vi "Get Console Reply(class).vi"(8 "error in (no error)":errorcluster, 11 "EditPanel API in":refnum<class "EditPanel API.lvclass">) -> (0 "error out":errorcluster, 2 "EditPanel API.lvlib:Console Reply.lvclass":refnum<class "Console Reply.lvclass">, 3 "EditPanel API out":refnum<class "EditPanel API.lvclass">)   [LabVIEW 2015, in "EditPanel API.lvlib" / "EditPanel API.lvclass"]
uses:
  EditPanel API.lvclass
  Console Reply/Console Reply/Console Reply.lvclass
  EditPanel API.lvclass/EditPanel API.ctl
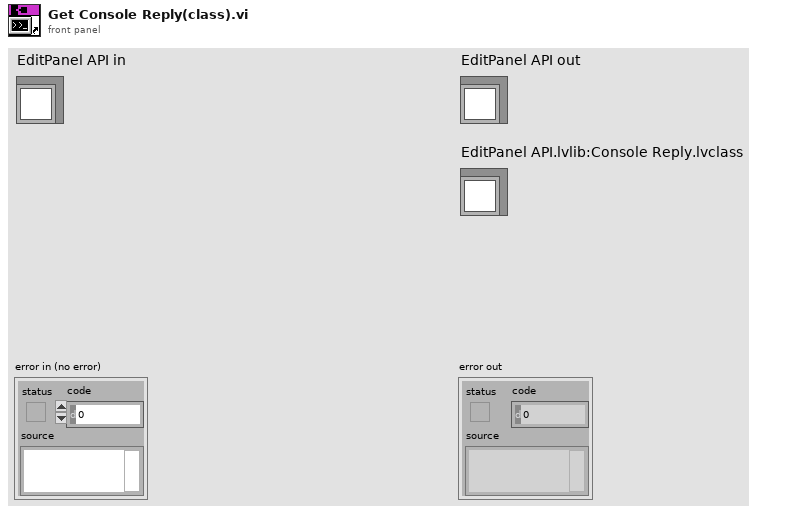
[diagram p1: front panel]
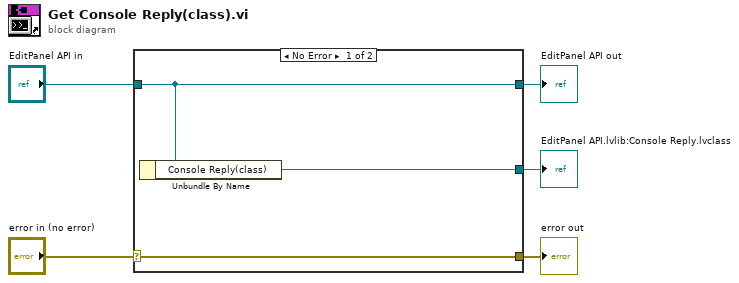
[diagram p0: block diagram]
diagram:
  n1 = case shown="No Error" "error in (no error)" {
    selector: "error in (no error)" -> [w8 w9]
    tunnel: [w8 w9] -> w4
    tunnel: [w7 w10] -> w2
    tunnel: "EditPanel API in" -> [w7 w10]
    tunnel: [w6 _] -> w1
    frame No Error {
      n2 = Unbundle By Name(w7) -> ("Console Reply(class)"=w6:refnum<class "Console Reply.lvclass">)
    }
    frame Error {
    }
  }
  "error out" <- w4
  "EditPanel API out" <- w2
  "EditPanel API.lvlib:Console Reply.lvclass" <- w1
